vi "Error Messages.vi"(0 "Device ID":T1(ring), 5 "Error Code":i32 format="%x", 11 "error in (no error)":errorcluster) -> (15 "error out":errorcluster)   [LabVIEW 2010]
doc: "This VI converts an error code number from the Robo Interface DLL into a string and creates an error cluster with this information."
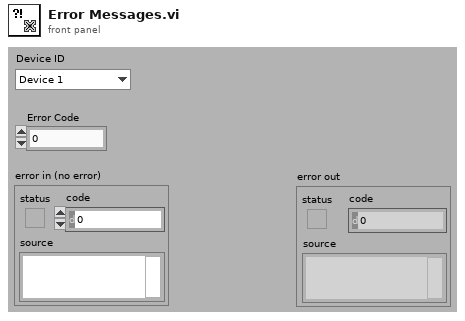
[diagram p1: front panel]
types:
  T1 = enum16{"Device 1", "Device 2", "Device 3", "Device 4", "Device 5", "Device 6", "Device 7", "Device 8"}
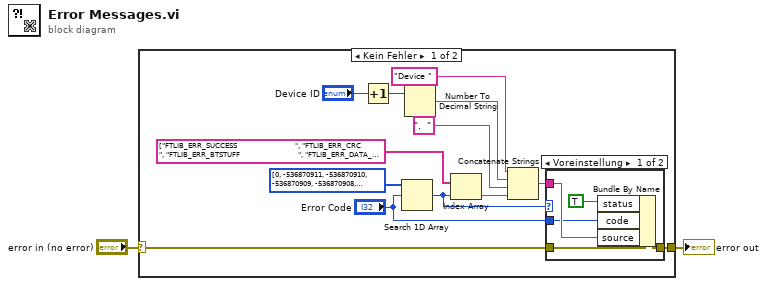
[diagram p0: block diagram]
diagram:
  n1 = case shown="Kein Fehler" "error in (no error)" {
    selector: "error in (no error)" -> [w12 w22]
    tunnel: [w11 w22] -> w1
    frame No Error {
      n2 = Increment(x="Device ID") -> (x+1=w3:T1)
      n3 = Search 1D Array(1D array=i32[] [0, -536870911, -536870910, -536870909, -536870908, -536870907, -536870906, -536870905, -536870904, -536870903, -536870902, -536870901, -536870900, -536870899, -536870897, -536870896, -536870895, -536870894, -536870893, -536870864, -536870656, -536870400, -536870144, -536869888, -536869376, -536869120, -536868864, -536868608, -536868352, -536868096, -536867840, -536867584, -536867328, -536867072, -402649088, -536862720, -536858624, -536854528, -536850432, -536846336, -536842240, -536838144, -536805376, -536739840, -536674304, -536608768, -536543232, -536866816, -536866815, -536866814, -536866813, -536866812, -536866811, -536866810, -536866809, -536866808, -536866807, -536866806, -536866805, -536866804, -536866803, -536866802, -536866801, -536866800, -536866799, -536866798, -536866797, -536866796, -536866795, -536866794, -536866793, -536866792, -536866790, -536866789, -536866788, -536866787, -536866688, -536866687, -536866686, -536866685, -536866684, -536866683, -536866682, -536866681, -536866560, -536866559, -536866558, -536866557, -536866556, -536866555, -536866554, -536866553, -536866552, -536866175, -536866174, -536866173, -536866172, -536866171, -536866170, -536866169, -536866168, -536866167, -536866166, -536866165, -536866160, -536866159, -536866158, -536866157, -536866155, -536866144, -536866143, -536866142, -536866141, -536866140, -536866139, -536866138, -536866137, -536866136, -536866135, -536866134, -536866133, -536866132, -536866131, -536866130, -536866112, -536866111, -536866110, -536866109, -536866108, -536866107, -536866106, -536866105, -536866104, -536866103, -536866102, -536866101, -536866099, -536866080, -536866079, -536866078, -536866077, -536866076, -536866075, -536866074, -536866073, -536866072, -536866071, -536865280, -536865279, -536865278, -536865248, -536864768, -536864767, -536864766, -536864765, -536864512, -536864511, -536864510, -536864509, -536864508, -536864507, -536864506, -536864505, -536864504, -536864503, -536864502, -536864501, -536864500, -536864499, -536864256, -536864255, -536864254, -536864253, -536864252, -536864251, -536864250, -536864248, -536864247, -536864246, -536864243, -536864242, -536864000, -536863999, -536863744, -536863743, -536863488, -536862976, -536862975, -536862974, -536862973, -536862972, -536862971, -536862970, -536862969, -536862968, -536862967, -536862966, -536862965, -536862964, -536862963, -536862962, -536862961, -536862768, -536862767, -536862766, -536862765, -536862764, -536862763, -536862762, -536862761, -536862760, -536862759, -536862758, -536862757, -536862756, -536862755, -536862754, -536862753, -536862752, -536862751, -536862750, -536862749, -536862748, -536862747, -536862746, -536862745, -536862744, -536862743, -536862742, -536862741, -536862740, -536862739, -536862738, -536862737, -536862736, -536862735, -536862734, -536862733, -536862732, -536862731, -536862730, -536862729, -536862728, -536862727, -536862726, -536862725, -536862724, -536862723, -536862722, -536862721] ("number"), element="Error Code") -> (index of element=w13:i32)  [unwired: 1 out]
      n4 = Number To Decimal String(number=w3) -> (decimal integer string=w8:string)  [unwired: 1 out]
      n5 = Index Array(array=string[] ["FTLIB_ERR_SUCCESS                             ", "FTLIB_ERR_CRC                                 ", "FTLIB_ERR_BTSTUFF                             ", "FTLIB_ERR_DATA_TOGGLE_MISMATCH                ", "FTLIB_ERR_STALL_PID                           ", "FTLIB_ERR_DEV_NOT_RESPONDING                  ", "FTLIB_ERR_PID_CHECK_FAILURE                   ", "FTLIB_ERR_UNEXPECTED_PID                      ", "FTLIB_ERR_DATA_OVERRUN                        ", "FTLIB_ERR_DATA_UNDERRUN                       ", "FTLIB_ERR_RESERVED1                           ", "FTLIB_ERR_RESERVED2                           ", "FTLIB_ERR_BUFFER_OVERRUN                      ", "FTLIB_ERR_BUFFER_UNDERRUN                     ", "FTLIB_ERR_NOT_ACCESSED                        ", "FTLIB_ERR_FIFO                                ", "FTLIB_ERR_XACT_ERROR                          ", "FTLIB_ERR_BABBLE_DETECTED                     ", "FTLIB_ERR_DATA_BUFFER_ERROR                   ", "FTLIB_ERR_ENDPOINT_HALTED                     ", "FTLIB_ERR_NO_MEMORY                           ", "FTLIB_ERR_INVALID_URB_FUNCTION                ", "FTLIB_ERR_INVALID_PARAMETER                   ", "FTLIB_ERR_ERROR_BUSY                          ", "FTLIB_ERR_INVALID_PIPE_HANDLE                 ", "FTLIB_ERR_NO_BANDWIDTH                        ", "FTLIB_ERR_INTERNAL_HC_ERROR                   ", "FTLIB_ERR_ERROR_SHORT_TRANSFER                ", "FTLIB_ERR_BAD_START_FRAME                     ", "FTLIB_ERR_ISOCH_REQUEST_FAILED                ", "FTLIB_ERR_FRAME_CONTROL_OWNED                 ", "FTLIB_ERR_FRAME_CONTROL_NOT_OWNED             ", "FTLIB_ERR_NOT_SUPPORTED                       ", "FTLIB_ERR_INVALID_CONFIGURATION_DESCRIPTOR    ", "FTLIB_ERR_INSUFFICIENT_RESOURCES              ", "FTLIB_ERR_SET_CONFIG_FAILED                   ", "FTLIB_ERR_USBD_BUFFER_TOO_SMALL               ", "FTLIB_ERR_USBD_INTERFACE_NOT_FOUND            ", "FTLIB_ERR_INVALID_PIPE_FLAGS                  ", "FTLIB_ERR_USBD_TIMEOUT                        ", "FTLIB_ERR_DEVICE_GONE                         ", "FTLIB_ERR_STATUS_NOT_MAPPED                   ", "FTLIB_ERR_CANCELED                            ", "FTLIB_ERR_ISO_NOT_ACCESSED_BY_HW              ", "FTLIB_ERR_ISO_TD_ERROR                        ", "FTLIB_ERR_ISO_NA_LATE_USBPORT                 ", "FTLIB_ERR_ISO_NOT_ACCESSED_LATE               ", "FTLIB_ERR_FAILED                              ", "FTLIB_ERR_INVALID_INBUFFER                    ", "FTLIB_ERR_INVALID_OUTBUFFER                   ", "FTLIB_ERR_OUT_OF_MEMORY                       ", "FTLIB_ERR_PENDING_REQUESTS                    ", "FTLIB_ERR_ALREADY_CONFIGURED                  ", "FTLIB_ERR_NOT_CONFIGURED                      ", "FTLIB_ERR_OPEN_PIPES                          ", "FTLIB_ERR_ALREADY_BOUND                       ", "FTLIB_ERR_NOT_BOUND                           ", "FTLIB_ERR_DEVICE_NOT_PRESENT                  ", "FTLIB_ERR_CONTROL_NOT_SUPPORTED               ", "FTLIB_ERR_TIMEOUT                             ", "FTLIB_ERR_INVALID_RECIPIENT                   ", "FTLIB_ERR_INVALID_TYPE                        ", "FTLIB_ERR_INVALID_IOCTL                       ", "FTLIB_ERR_INVALID_DIRECTION                   ", "FTLIB_ERR_TOO_MUCH_ISO_PACKETS                ", "FTLIB_ERR_POOL_EMPTY                          ", "FTLIB_ERR_PIPE_NOT_FOUND                      ", "FTLIB_ERR_INVALID_ISO_PACKET                  ", "FTLIB_ERR_OUT_OF_ADDRESS_SPACE                ", "FTLIB_ERR_INTERFACE_NOT_FOUND                 ", "FTLIB_ERR_INVALID_DEVICE_STATE                ", "FTLIB_ERR_INVALID_PARAM                       ", "FTLIB_ERR_INVALID_POWER_STATE                 ", "FTLIB_ERR_POWER_DOWN                          ", "FTLIB_ERR_VERSION_MISMATCH                    ", "FTLIB_ERR_SET_CONFIGURATION_FAILED            ", "FTLIB_ERR_VID_RESTRICTION                     ", "FTLIB_ERR_ISO_RESTRICTION                     ", "FTLIB_ERR_BULK_RESTRICTION                    ", "FTLIB_ERR_EP0_RESTRICTION                     ", "FTLIB_ERR_PIPE_RESTRICTION                    ", "FTLIB_ERR_PIPE_SIZE_RESTRICTION               ", "FTLIB_ERR_CONTROL_RESTRICTION                 ", "FTLIB_ERR_INTERRUPT_RESTRICTION               ", "FTLIB_ERR_DEVICE_NOT_FOUND                    ", "FTLIB_ERR_SOME_DEVICES_ARE_OPEN               ", "FTLIB_ERR_DEVICE_IS_OPEN                      ", "FTLIB_ERR_DEVICE_NOT_OPEN                     ", "FTLIB_ERR_NO_SUCH_DEVICE_INSTANCE             ", "FTLIB_ERR_INVALID_FUNCTION_PARAM              ", "FTLIB_ERR_DESTROY_DEVICE_LIST                 ", "FTLIB_ERR_USB_NOT_SUPPORTET_FROM_OS           ", "FTLIB_ERR_CLOSE_DEVICE                        ", "FTLIB_ERR_DEVICE_NOT_SUPPORTET                ", "FTLIB_ERR_WRONG_DEVICE_NUMBER                 ", "FTLIB_ERR_UNKNOWN_DEVICE_HANDLE               ", "FTLIB_ERR_WRONG_USB_HANDLE                    ", "FTLIB_ERR_WRONG_PATHNAME                      ", "FTLIB_ERR_LIB_IS_INITIALIZED                  ", "FTLIB_ERR_LIB_IS_NOT_INITIALIZED              ", "FTLIB_ERR_SERIAL_NR_UNKNOWN                   ", "FTLIB_ERR_POWER_TOO_LOW                       ", "FTLIB_ERR_WRONG_RETURN_VALUE                  ", "FTLIB_ERR_USB_SUPPORT_IS_NOT_INITIALIZED      ", "FTLIB_ERR_USB_MUT0                            ", "FTLIB_ERR_USB_MUT1                            ", "FTLIB_ERR_USB_MUT2                            ", "FTLIB_ERR_USB_MUT3                            ", "FTLIB_ERR_USB_DEVICE_IS_IN_USE                ", "FTLIB_ERR_THREAD_NOT_STARTABLE                ", "FTLIB_ERR_THREAD_NOT_STARTABLE_X1             ", "FTLIB_ERR_THREAD_NOT_STARTABLE_X2             ", "FTLIB_ERR_THREAD_NOT_STARTABLE_X3             ", "FTLIB_ERR_OTHER_THREAD_FOR_SAME_DEVICE_IS_RUN ", "FTLIB_ERR_THREAD_IS_RUNNING                   ", "FTLIB_ERR_THREAD_NOT_RUNNING                  ", "FTLIB_ERR_THREAD_X1                           ", "FTLIB_ERR_THREAD_X2                           ", "FTLIB_ERR_THREAD_WRITE_USB                    ", "FTLIB_ERR_THREAD_READ_USB                     ", "FTLIB_ERR_THREAD_IS_NORMAL_STOPPED            ", "FTLIB_ERR_THREAD_WAIT_TIMEOUT                 ", "FTLIB_ERR_THREAD_WRITE_COM                    ", "FTLIB_ERR_THREAD_READ_COM                     ", "FTLIB_ERR_DOWNLOAD                            ", "FTLIB_ERR_DOWNLOAD_WRONG_PARAMETER            ", "FTLIB_ERR_DOWNLOAD_WRONG_MEM_BLOCK            ", "FTLIB_ERR_DOWNLOAD_DATA_SIZE_IS_NULL          ", "FTLIB_ERR_DOWNLOAD_DATA_SIZE_TOO_BIG          ", "FTLIB_ERR_DOWNLOAD_DATA_SIZE                  ", "FTLIB_ERR_DOWNLOAD_ERASE                      ", "FTLIB_ERR_DOWNLOAD_F5                         ", "FTLIB_ERR_DOWNLOAD_PROG_SNF1                  ", "FTLIB_ERR_DOWNLOAD_PROG_SNF2                  ", "FTLIB_ERR_DOWNLOAD_BLOCK                      ", "FTLIB_ERR_DOWNLOAD_BLOCK_NR                   ", "FTLIB_ERR_DOWNLOAD_CRC                        ", "FTLIB_ERR_IF_NO_PROGRAM                       ", "FTLIB_ERR_IF_PROGRAM_IS_RUNNING               ", "FTLIB_ERR_IF_NO_PROGRAM_IS_RUNNING            ", "FTLIB_ERR_IF_WRONG_PROG_NUMBER                ", "FTLIB_ERR_IF_BUFFER_TOO_SMALL                 ", "FTLIB_ERR_IF_MEM_ADDRESS                      ", "FTLIB_ERR_IF_MEM_VERIFY                       ", "FTLIB_ERR_IF_NOT_SUPPORTET_MODUS              ", "FTLIB_ERR_IF_FUNCTION_NOT_SUPPORT             ", "FTLIB_ERR_FUNCTION_OVER_RF_NOT_ALLOWED        ", "FTLIB_INFO_PROGRAM_0_IS_RUNNING               ", "FTLIB_INFO_PROGRAM_1_IS_RUNNING               ", "FTLIB_INFO_PROGRAM_2_IS_RUNNING               ", "FTLIB_INFO_ONLINE_MODUS                       ", "FTLIB_FIRMWARE_UPDATE_FILE_WRONG_0            ", "FTLIB_FIRMWARE_UPDATE_CRC                     ", "FTLIB_FIRMWARE_UPDATE_FILE_OLD                ", "FTLIB_FIRMWARE_UPDATE_FILE_WRONG_1            ", "FTLIB_ERR_PORT_NUMBER                         ", "FTLIB_ERR_WRONG_PORT                          ", "FTLIB_ERR_PORT_NUMBER_IS_NULL                 ", "FTLIB_ERR_TYP                                 ", "FTLIB_ERR_PORT_NOT_FOUND                      ", "FTLIB_ERR_ACCESS_DENIED                       ", "FTLIB_ERR_OPEN_COM                            ", "FTLIB_ERR_CLOSE_COM                           ", "FTLIB_ERR_INIT_COM                            ", "FTLIB_ERR_INIT_COM_TIMEOUT                    ", "FTLIB_ERR_WRITE_COM                           ", "FTLIB_ERR_READ_COM                            ", "FTLIB_ERR_READ_COM_NUMBER                     ", "FTLIB_ERR_READ_COM_NOTHING                    ", "FTLIB_ERR_RF_NOT_INSTALLED                    ", "FTLIB_ERR_RF_WRONG_CHANNEL                    ", "FTLIB_ERR_RF_WRONG_SUB_CHANNEL                ", "FTLIB_ERR_RF_NO_CONNECTION                    ", "FTLIB_ERR_RF_NO_CONNECTION_A                  ", "FTLIB_ERR_RF_NO_CONNECTION_B                  ", "FTLIB_ERR_RF_NO_CONNECTION_C                  ", "FTLIB_ERR_RF_TIMEOUT_1                        ", "FTLIB_ERR_RF_TIMEOUT_2                        ", "FTLIB_ERR_RF_FW_OLD1                          ", "FTLIB_ERR_RF_INTERNAL_1                       ", "FTLIB_ERR_RF_NO_INTERFACE_MODULE_FOUND        ", "FTLIB_ERR_DLL_NOT_LOADABLE                    ", "FTLIB_ERR_DLL_FUNCTION_ERROR                  ", "FTLIB_ERR_MSG_HWID_WRONG                      ", "FTLIB_ERR_MSG_BUFFER_FULL_TIMEOUT             ", "FTLIB_ERR_UNKNOWN_OPTION_VALUE                ", "FTLIB_ERR_INTERFACE_00                        ", "FTLIB_ERR_INTERFACE_01                        ", "FTLIB_ERR_INTERFACE_02                        ", "FTLIB_ERR_INTERFACE_03                        ", "FTLIB_ERR_INTERFACE_04                        ", "FTLIB_ERR_INTERFACE_05                        ", "FTLIB_ERR_INTERFACE_06                        ", "FTLIB_ERR_INTERFACE_07                        ", "FTLIB_ERR_INTERFACE_08                        ", "FTLIB_ERR_INTERFACE_09                        ", "FTLIB_ERR_INTERFACE_0A                        ", "FTLIB_ERR_INTERFACE_0B                        ", "FTLIB_ERR_INTERFACE_0C                        ", "FTLIB_ERR_INTERFACE_0D                        ", "FTLIB_ERR_INTERFACE_0E                        ", "FTLIB_ERR_INTERFACE_0F                        ", "FTLIB_ERR_INTERFACE_D0                        ", "FTLIB_ERR_INTERFACE_D1                        ", "FTLIB_ERR_INTERFACE_D2                        ", "FTLIB_ERR_INTERFACE_D3                        ", "FTLIB_ERR_INTERFACE_D4                        ", "FTLIB_ERR_INTERFACE_D5                        ", "FTLIB_ERR_INTERFACE_D6                        ", "FTLIB_ERR_INTERFACE_D7                        ", "FTLIB_ERR_INTERFACE_D8                        ", "FTLIB_ERR_INTERFACE_D9                        ", "FTLIB_ERR_INTERFACE_DA                        ", "FTLIB_ERR_INTERFACE_DB                        ", "FTLIB_ERR_INTERFACE_DC                        ", "FTLIB_ERR_INTERFACE_DD                        ", "FTLIB_ERR_INTERFACE_DE                        ", "FTLIB_ERR_INTERFACE_DF                        ", "FTLIB_ERR_INTERFACE_E0                        ", "FTLIB_ERR_INTERFACE_E1                        ", "FTLIB_ERR_INTERFACE_E2                        ", "FTLIB_ERR_INTERFACE_E3                        ", "FTLIB_ERR_INTERFACE_E4                        ", "FTLIB_ERR_INTERFACE_E5                        ", "FTLIB_ERR_INTERFACE_E6                        ", "FTLIB_ERR_INTERFACE_E7                        ", "FTLIB_ERR_INTERFACE_E8                        ", "FTLIB_ERR_INTERFACE_E9                        ", "FTLIB_ERR_INTERFACE_EA                        ", "FTLIB_ERR_INTERFACE_EB                        ", "FTLIB_ERR_INTERFACE_EC                        ", "FTLIB_ERR_INTERFACE_ED                        ", "FTLIB_ERR_INTERFACE_EE                        ", "FTLIB_ERR_INTERFACE_EF                        ", "FTLIB_ERR_INTERFACE_F0                        ", "FTLIB_ERR_INTERFACE_F1                        ", "FTLIB_ERR_INTERFACE_F2                        ", "FTLIB_ERR_INTERFACE_F3                        ", "FTLIB_ERR_INTERFACE_F4                        ", "FTLIB_ERR_INTERFACE_F5                        ", "FTLIB_ERR_INTERFACE_F6                        ", "FTLIB_ERR_INTERFACE_F7                        ", "FTLIB_ERR_INTERFACE_F8                        ", "FTLIB_ERR_INTERFACE_F9                        ", "FTLIB_ERR_INTERFACE_FA                        ", "FTLIB_ERR_INTERFACE_FB                        ", "FTLIB_ERR_INTERFACE_FC                        ", "FTLIB_ERR_INTERFACE_FD                        ", "FTLIB_ERR_INTERFACE_FE                        ", "FTLIB_ERR_INTERFACE_FF                        "] ("Array 2"), index=w13) -> (element=w5:string)
      n6 = Concatenate Strings("Device " ("string"), w8, ".  " ("string"), w5) -> (w4:string)
      n7 = case shown="Voreinstellung" w13 {
        tunnel: w4 -> [w18 _]
        tunnel: w12 -> [w20 w21]
        tunnel: [w17 w21] -> w11
        tunnel: "Error Code" -> [w16 _]
        frame Default {
          n8 = Bundle By Name(cluster=w20, "status"=TRUE, "code"=w16, "source"=w18) -> (w17:errorcluster)
        }
        frame -1, 0 {
        }
      }
    }
    frame Error {
    }
  }
  "error out" <- w1
